vi "smartWatch.vi"() -> ()   [LabVIEW 2019]
panel:
  in  ".NET Container":refnum<k24>(container)
  in  "Tab Control":enum32{"Page 1", "Page 2"}(tab)
  out "Minutes":dbl
  out "Seconds":dbl
  out "Hours":dbl
  in  "stop":bool
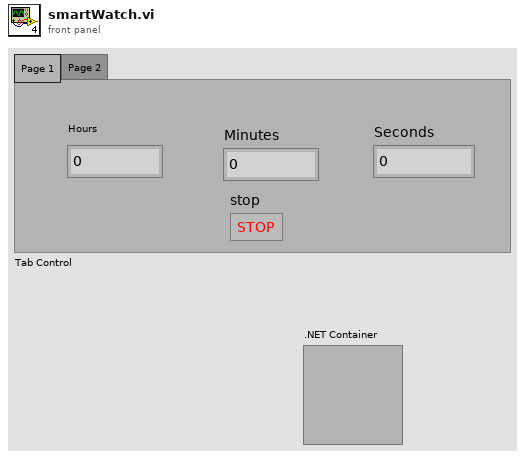
[diagram p1: front panel]
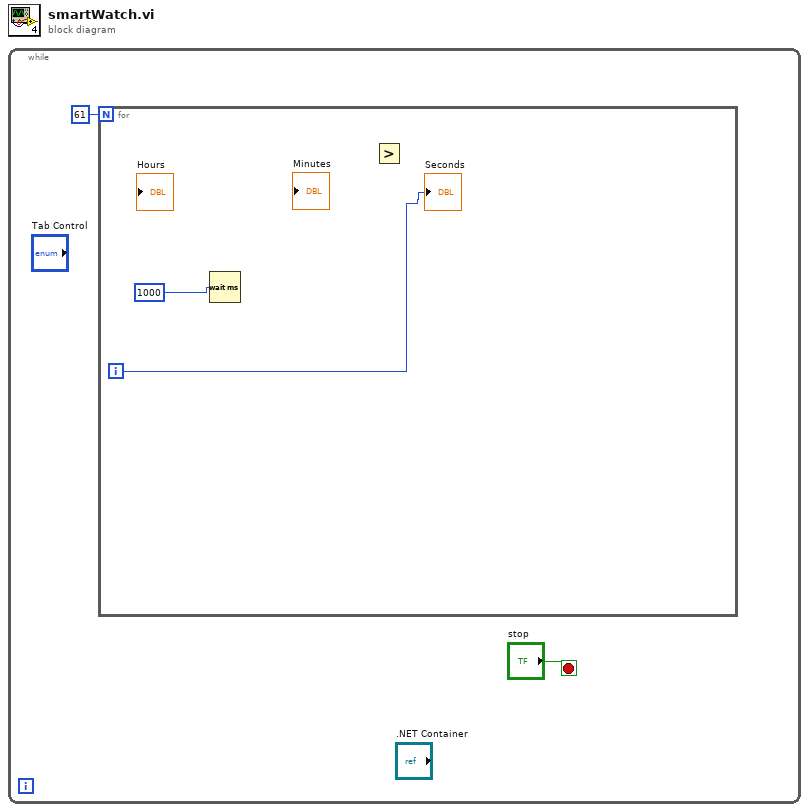
[diagram p0: block diagram]
diagram:
  n1 = while {
    stop <- "stop" stop-if-true
    n2 = for {
      N: 61 -> [_]
      i -> [w4]
      n3 = Wait (ms)(milliseconds to wait=u32 1000 ("millisecond timer value")) -> ()  [unwired: 1 out]
      n4 = Greater?() -> ()  [unwired: 2 in, 1 out]
      "Seconds" <- w4
    }
  }
